vi "Test Save PNG (Path).vi"(8 "error in (no error)":errorcluster) -> (0 "error out":errorcluster, 3 "Pass?":bool)   [LabVIEW 2020]
uses:
  <vilib>/picture/picture.llb/imagedata.ctl
  G-Image/Image IO/Polymorphic VIs/Load Image (Path).vi
  G-Image/G-Image.lvlib
  G-Image/Image IO/Polymorphic VIs/Save PNG Image (Path).vi
panel:
  out "Array":cluster{string, "new picture":picture}[](array[cluster])
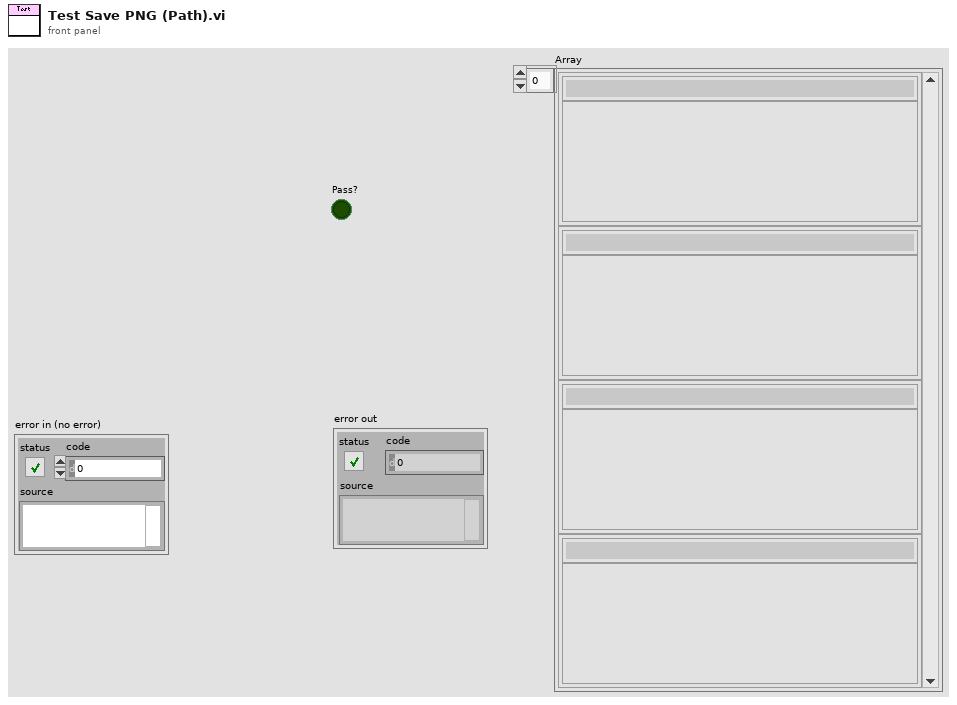
[diagram p1: front panel]
types:
  T1 = typedef "imagedata.ctl" = cluster{"image type":i32, "image depth":i32, "image":u8[], "mask":u8[], "colors":u32[], "Rectangle":cluster{"left":i16, "top":i16, "right":i16, "bottom":i16}}
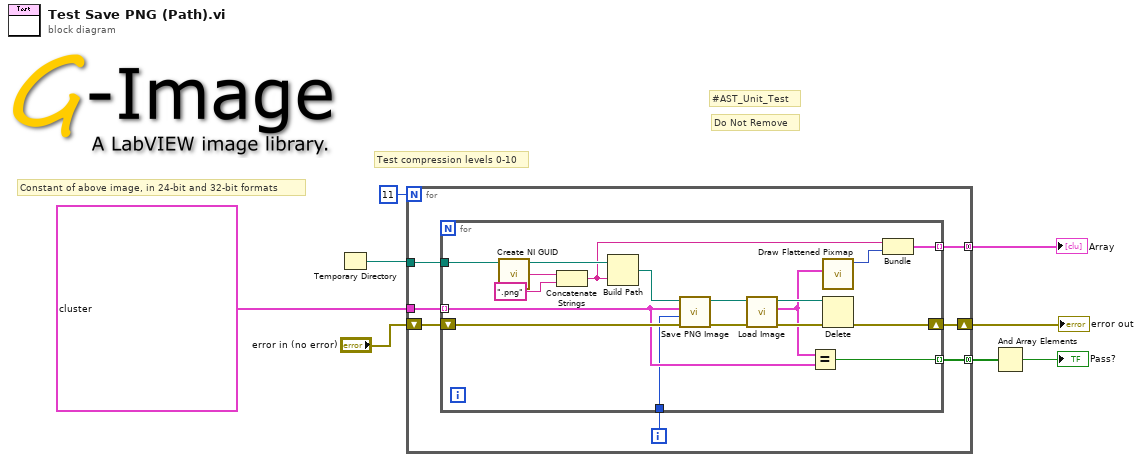
[diagram p0: block diagram]
diagram:
  # "Test compression levels 0-10"
  # "Constant of above image, in 24-bit and 32-bit formats"
  # "Do Not Remove"
  # "#AST_Unit_Test"
  n1 = Temporary Directory() -> (w7:path)
  n2 = for {
    N: 11 -> [_]
    tunnel: w7 -> [w14]
    tunnel: [w13] -> w6 mode=concatenating
    tunnel: [w11] -> w4 mode=concatenating
    tunnel: T1[] [{"image type"=0, "image depth"=24, "image"=array[115500 elements], "mask"=[], "colors"=[], "Rectangle"={"left"=0, "top"=0, "right"=350, "bottom"=110}}, {"image type"=0, "image depth"=32, "image"=array[154000 elements], "mask"=array[4840 elements], "colors"=[], "Rectangle"={"left"=0, "top"=0, "right"=350, "bottom"=110}}] ("Array 2") -> [w10]
    shift-right: [w12] -> w5
    shift-left: "error in (no error)" -> [w15]
    i -> [w9]
    n3 = for {
      tunnel: w14 -> [w29]
      tunnel: w10 -> [w25] mode=indexing
      shift-right: [w22] -> w12
      shift-left: w15 -> [w32]
      tunnel: [w21] -> w11 mode=indexing
      tunnel: [w17] -> w13 mode=indexing
      tunnel: w9 -> [w16]
      n4 = call <vilib>:"Create NI GUID.vi"() -> ("NI GUID"=w30:string)
      n5 = Concatenate Strings(w30, ".png" ("string")) -> (w18:string)
      n6 = Build Path(base path=w29, name or relative path=w18) -> (appended path=w28:path)
      n7 = call-poly "Save PNG Image.vi"("error in (no error)"=w32, "Compression (6)"=w16, "Image"=w25, "Path In"=w28) -> ("error out"=w26:errorcluster, "Path Out"=w27:path)  [unwired: 6 in]
      n8 = call-poly "Load Image.vi"("error in (no error)"=w26, "Path In"=w27) -> ("error out"=w23:errorcluster, "Image"=w20:T1, "Path Out"=w24:path)  [unwired: 7 in]
      n9 = Equal?(x=w20, y=w25) -> (x = y?=w21:bool)
      n10 = call <vilib>:"Draw Flattened Pixmap.vi"("image data"=w20) -> ("new picture"=w19:picture)  [unwired: 8 in]
      n11 = Delete(path (use dialog)=w24, error in=w23) -> (error out=w22:errorcluster)  [unwired: 3 in, 2 out]
      n12 = Bundle(w18, "new picture"=w19) -> (w17:cluster{string, "new picture":picture})  [unwired: 1 in]
    }
  }
  "error out" <- w5
  "Array" <- w6
  n13 = And Array Elements(Boolean array=w4) -> (logical AND=→"Pass?":bool)
